vi "SplashWnd - Module Starting Up3.vi"(5 "Background VI Ref (Callee's Caller)":refnum<vi>, 6 "LoadingWait(ms)":u32=100, 7 "Title":string, 8 "Error In (No Error)":errorcluster, 9 "Name (\"\" to Use UUID)":string="SplashWindow") -> (0 "error out":errorcluster)   [LabVIEW 2020]
uses:
  csm/CSM-Utils/CSM-ModuleManager/Operation.ctl
  79d02799-5e27-450a-8f22-22593f2d7556.vi
  csm/CSM-ModSets-SplashWindow/SplashWindow.vi
  <userlib>/_NEVSTOP/Communicable State Machine(CSM)/addons/API-String-Arugments-Support/_Support/Data To API String Arguments.vi
  csm/CSM-ModSets-SplashWindow/CSM-SplashWindow.lvlib
  <userlib>/_NEVSTOP/Communicable State Machine(CSM)/Communicable State Machine.lvlib
  <userlib>/_NEVSTOP/Communicable State Machine(CSM)/addons/INI-Static-Variable-Support/INI-Static-Variable-Support.lvlib
  csm/CSM-Utils/CSM-ModuleManager/CSM-ModuleManager.lvlib
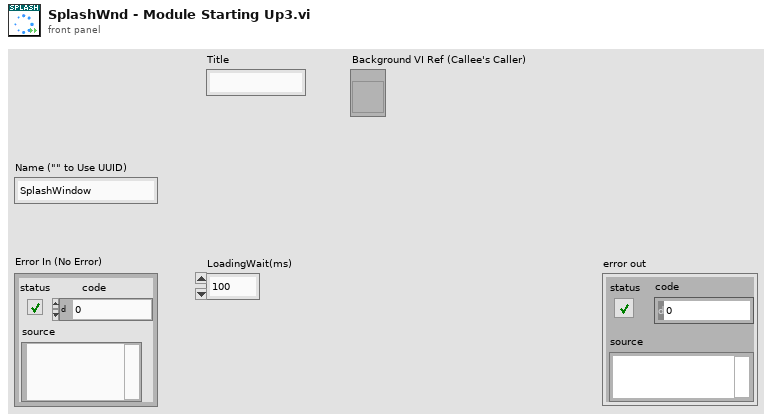
[diagram p1: front panel]
types:
  T1 = typedef "CSM-ModuleManager.lvlib/Operation.ctl" = enum16{"Register", "UnRegister", "Load Config", "Get"}
  T2 = enum32{"Invalid", "Default", "Floating", "Floating/Auto-Hide", "Modal"}
  T3 = enum32{"Invalid", "Standard", "Closed", "Hidden", "Minimized", "Maximized"}
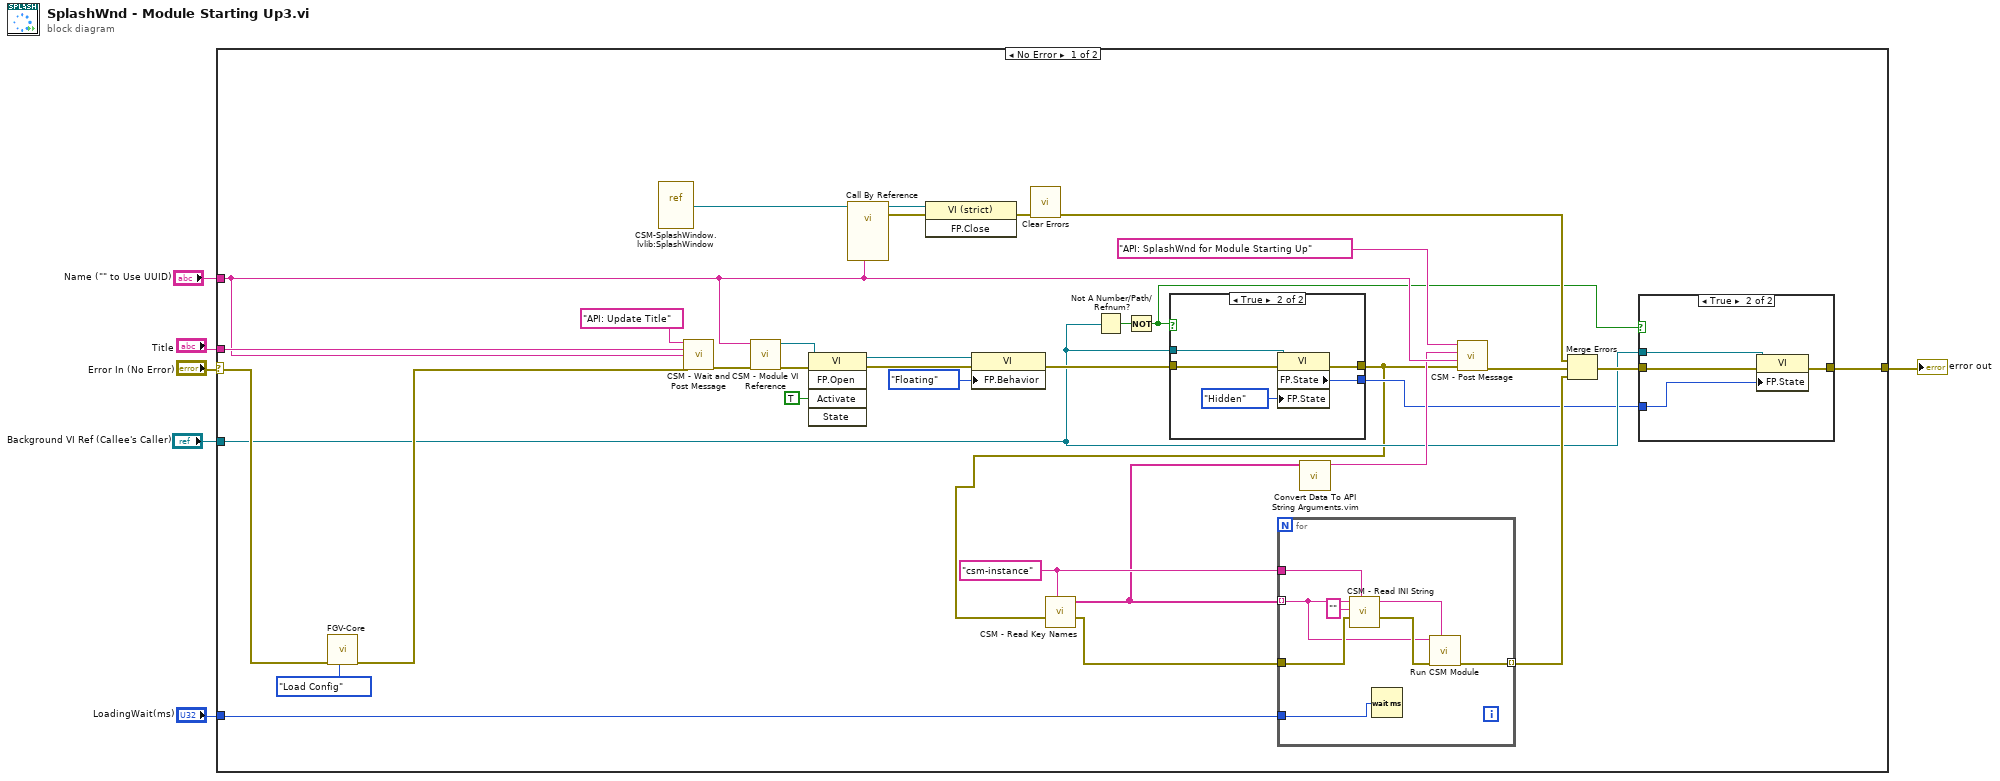
[diagram p0: block diagram]
diagram:
  n1 = case shown="No Error" "Error In (No Error)" {
    selector: "Error In (No Error)" -> [w21 w60]
    tunnel: "Title" -> [w40 _]
    tunnel: [w13 w60] -> w4
    tunnel: "Name (\"\" to Use UUID)" -> [w39 _]
    tunnel: "Background VI Ref (Callee's Caller)" -> [w11 _]
    tunnel: "LoadingWait(ms)" -> [w9 _]
    frame No Error {
      w22 = "csm-instance" ("Section Name (\"\" as Default)")
      n2 = call "FGV-Core.vi"("Enum"=Operation."Load Config", "error in (no error)"=w21) -> ("error out"=w18:errorcluster)  [unwired: 7 in, 2 out]
      n3 = vi-ref "CSM-SplashWindow.lvlib:SplashWindow.vi"() -> (w17:refnum<vi>)
      n4 = call <userlib>:"CSM - Wait and Post Message.vi"("State"="API: Update Title", "Arguments (\"\")"=w40, "Target Module"=w39, "Error In (No Error)"=w18) -> ("error out"=w37:errorcluster)  [unwired: 10 in, 1 out]
      n5 = call <userlib>:"CSM - Module VI Reference.vi"("error in (no error)"=w37, "CSM Name"=w39) -> ("error out"=w35:errorcluster, "CSM Module VIRef"=w36:refnum<vi>)  [unwired: 8 in]
      n6 = invoke class="VI" method="FP.Open"(reference=w36, error in=w35, "Activate"=TRUE ("Activate?")) -> (reference out=w33:refnum<vi>, error out=w34:errorcluster)  [unwired: 2 in, 3 out]
      n7 = call-by-ref "?"(reference=w17, "Name (\"\" to Use UUID)"=w39) -> (reference out=w26:refnum<vi>, error out=w30:errorcluster)  [unwired: 12 in]
      n8 = invoke class="VI (strict)" method="FP.Close"(reference=w26, error in=w30) -> (error out=w27:errorcluster)  [unwired: 1 in, 2 out]
      n9 = property class="VI"(reference=w33, error in=w34, "FP.Behavior"=T2."Floating" ("Front Panel Window:Behavior")) -> (error out=w15:errorcluster)  [unwired: 1 out]
      n10 = call <vilib>:"Clear Errors.vi"("error in (no error)"=w27) -> ("error out"=w25:errorcluster)  [unwired: 5 in, 1 out]
      n11 = Not A Number/Path/Refnum?(number/path/refnum=w11) -> (NaN/Path/Refnum?=w16:bool)
      n12 = Not(x=w16) -> (.not. x?=w12:bool)
      n13 = case shown="True" w12 {
        tunnel: w15 -> [w46 w51]
        tunnel: [w46 w49] -> w7
        tunnel: w11 -> [_ w50]
        tunnel: [_ w47] -> w10
        frame False {
        }
        frame True {
          n14 = property class="VI"(reference=w50, error in=w51, "FP.State"=T3."Hidden" ("Front Panel Window:State")) -> (error out=w49:errorcluster, "FP.State"=w47:T3)  [unwired: 1 out]
        }
      }
      n15 = call <userlib>:"CSM - Read Key Names.vi"("Section Name (\"\" as Default)"=w22, "error in (no error)"=w7) -> ("error out"=w24:errorcluster, "Keys"=w20:string[])  [unwired: 6 in]
      n16 = for {
        tunnel: w22 -> [w58]
        tunnel: w20 -> [w53] mode=indexing
        tunnel: w24 -> [w59]
        tunnel: [w55] -> w19 mode=indexing
        tunnel: w9 -> [w52]
        n17 = call <userlib>:"CSM - Read INI String.vi"("Section Name (\"\" as Default)"=w58, "error in (no error)"=w59, "Default Value"="", "Variable Name"=w53) -> ("error out"=w56:errorcluster, "Value"=w54:string)  [unwired: 3 in, 1 out]
        n18 = Wait (ms)(milliseconds to wait=w52) -> ()  [unwired: 1 out]
        n19 = call "Run CSM Module.vi"("CSM-Module"=w54, "Error in"=w56, "CSM-Instance"=w53) -> ("Error out"=w55:errorcluster)  [unwired: 8 in]
      }
      n20 = call "Convert Data To API String Arguments.vim"("Data"=w20) -> ("API String"=w29:string)  [unwired: 7 in, 1 out]
      n21 = call <userlib>:"CSM - Post Message.vi"("Error In (No Error)"=w7, "Target Module"=w39, "Arguments (\"\")"=w29, "State"="API: SplashWnd for Module Starting Up") -> ("error out"=w8:errorcluster)  [unwired: 7 in]
      n22 = Merge Errors(w25, w8, w19) -> (w14:errorcluster)
      n23 = case shown="True" w12 {
        tunnel: w14 -> [w41 w45]
        tunnel: [w41 w43] -> w13
        tunnel: w11 -> [_ w44]
        tunnel: w10 -> [_ w42]
        frame False {
        }
        frame True {
          n24 = property class="VI"(reference=w44, error in=w45, "FP.State"=w42) -> (error out=w43:errorcluster)  [unwired: 1 out]
        }
      }
    }
    frame Error {
    }
  }
  "error out" <- w4
